vi "Add Monitor Recorders.vi"(6 "Reset":bool, 8 "error in (no error)":errorcluster, 10 "Module type":T1, 11 "Monitor-Pulse in":refnum<class "Application Controller.lvclass">) -> (0 "error out":errorcluster, 2 "Actot names out":string[](array[string]), 3 "Monitor-Pulse out":refnum<class "Application Controller.lvclass">)   [LabVIEW 2018, in "Application Controller.lvclass"]
uses:
  Application Controller.lvclass
  Module Types.ctl
  Instrument Actor/Instrument Actor.lvclass
  C:/github/2018/LabActor/Worker/Worker.lvclass
  Recorders/Micron Optics/Micron Optics Recorder.lvclass
  C:/github/2018/LabActor/Recorders/Spectrometer/Spectrometer.lvclass
  NHMFL_Core/Libraries/Instruments/Micron Optics/Micron Hyperion Driver/Micron Hyperion Driver.lvclass
  C:/github/2018/NHMFL_Core/Libraries/Instruments/Spectrometer Driver/Spectrometer Driver.lvclass
  Spectrum Recorder too/Spectrum Recorder too.lvclass
  C:/github/2018/LabActor/Instrument Actor/Instrument Actor.lvclass
  NHMFL_Core/Libraries/Red Pitaya/RP Core/Red Pitaya Transceiver Driver/Red Pitaya Transceiver Driver.lvclass
  C:/github/2018/NHMFL_Core/Libraries/Instruments/Instrument Driver/Instrument Driver.lvclass
  Instrument Actor/Instrument Actor.lvclass/Instrument Actor.ctl
  Post-Processors/Elastic Moduli/Format Resonances.lvclass
  Application Controller.lvclass/Application Controller.ctl
  Instrument Actor/Write Instrument driver.vi
  Read Monitor ref.vi
  Write Monitor ref.vi
  Worker/Worker.lvclass
  C:/github/2018/LabActor/Template Module/Template Module.lvclass
  Recorders/Spectrometer/Write Spectrometer Driver.lvclass.vi
  NHMFL_Core/Libraries/Queued Listbox/Queued Listbox.xctl
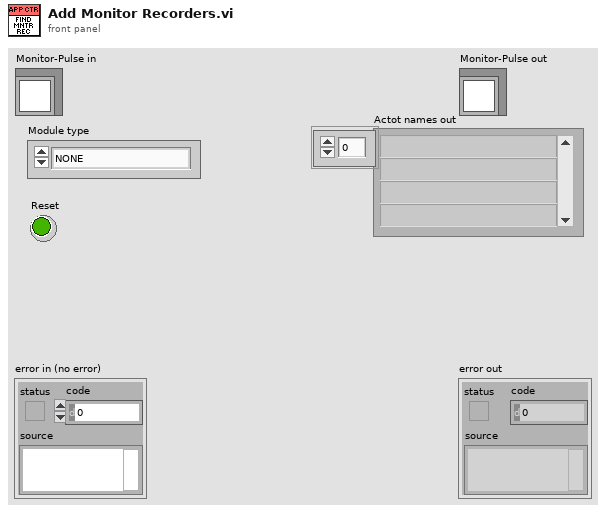
[diagram p1: front panel]
types:
  T1 = typedef "Module Types.ctl" = enum16{"NONE", "NI-DAQmx", "NI-Scope", "Red Pitaya Digitizer", "GaGe", "VISA Device", "Red Pitaya Lockin", "Monitor Controller", "Pulse Controller", "Integrate Pulse", "Lockin Processor", "File converter", "NHMFL Synthesizer", "Micron Hyperion", "Spectrum Recorder", "Resonance Detector", "TCP Communications", "Format Resonances", "Ruby Spectra", "PID Controller"}
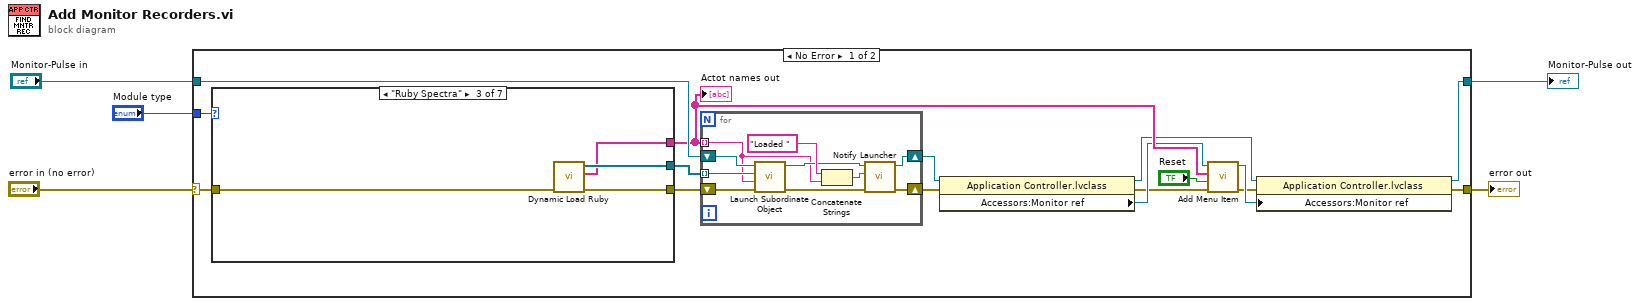
[diagram p0: block diagram]
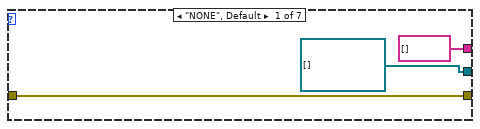
[diagram p2: hidden frame]
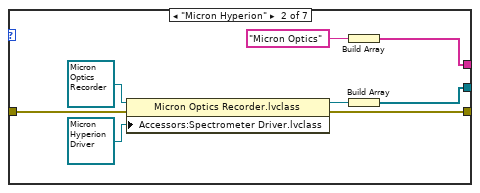
[diagram p3: hidden frame]
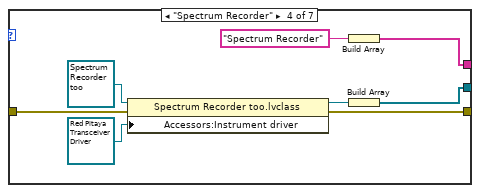
[diagram p4: hidden frame]
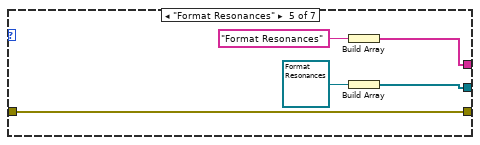
[diagram p5: hidden frame]
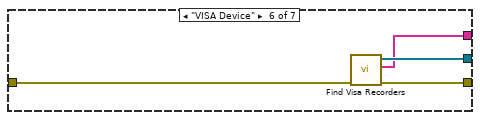
[diagram p6: hidden frame]
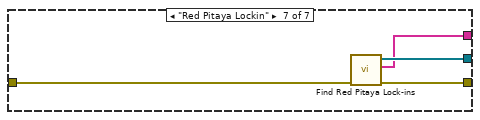
[diagram p7: hidden frame]
diagram:
  n1 = case shown="No Error" "error in (no error)" {
    selector: "error in (no error)" -> [w21 w69]
    tunnel: [w6 w69] -> w4
    tunnel: [w12 w68] -> w2
    tunnel: "Monitor-Pulse in" -> [w20 w68]
    tunnel: "Module type" -> [w17 _]
    frame No Error {
      n2 = case shown="\"Ruby Spectra\"" w17 {
        tunnel: w21 -> [w22 w31 w36 w43 w48 w53 w56]
        tunnel: [refnum<class "Instrument Actor.lvclass">[] [] ("Recorders List") w32 w34 w44 w49 w52 w55] -> w19
        tunnel: [string[] [] ("Names") w25 w33 w37 w45 w51 w54] -> w15
        tunnel: [w22 w30 w35 w42 w48 w50 w57] -> w18
        frame "NONE", Default {
        }
        frame "Micron Hyperion" {
          n3 = property class="Micron Optics Recorder.lvclass"(reference=refnum<class "Micron Optics Recorder.lvclass"> refnum ("Micron Optics Recorder.lvclass"), error in=w31, "Accessors:Spectrometer Driver.lvclass"=refnum<class "Micron Hyperion Driver.lvclass"> refnum ("Micron Hyperion Driver.lvclass")) -> (reference out=w28:refnum<class "Micron Optics Recorder.lvclass">, error out=w30:errorcluster)
          n4 = Build Array("Micron Optics") -> (w25:string[])
          n5 = Build Array(w28) -> (w32:refnum<class "Micron Optics Recorder.lvclass">[])
        }
        frame "Ruby Spectra" {
          n6 = call "Dynamic Load Ruby.vi"("Error In"=w36) -> ("Error Out"=w35:errorcluster, "Device names"=w33:string[], "Digitizers out"=w34:refnum<class "Instrument Actor.lvclass">[])  [unwired: 8 in]
        }
        frame "Spectrum Recorder" {
          n7 = property class="Spectrum Recorder too.lvclass"(reference=refnum<class "Spectrum Recorder too.lvclass"> refnum ("Spectrum Recorder too.lvclass"), error in=w43, "Accessors:Instrument driver"=refnum<class "Red Pitaya Transceiver Driver.lvclass"> refnum ("Red Pitaya Transceiver Driver.lvclass")) -> (reference out=w40:refnum<class "Spectrum Recorder too.lvclass">, error out=w42:errorcluster)
          n8 = Build Array("Spectrum Recorder") -> (w37:string[])
          n9 = Build Array(w40) -> (w44:refnum<class "Spectrum Recorder too.lvclass">[])
        }
        frame "Format Resonances" {
          n10 = Build Array("Format Resonances") -> (w45:string[])
          n11 = Build Array(refnum<class "Format Resonances.lvclass"> refnum ("Elastic Moduli.lvclass")) -> (w49:refnum<class "Format Resonances.lvclass">[])
        }
        frame "VISA Device" {
          n12 = call "Find Visa Recorders.vi"("Error In"=w53) -> ("Error Out"=w50:errorcluster, "Names"=w51:string[], "Recorders List"=w52:refnum<class "Instrument Actor.lvclass">[])  [unwired: 8 in]
        }
        frame "Red Pitaya Lockin" {
          n13 = call "Find Red Pitaya Lock-ins.vi"("Error In"=w56) -> ("Error Out"=w57:errorcluster, "Names"=w54:string[], "Instruments out"=w55:refnum<class "Instrument Actor.lvclass">[])  [unwired: 7 in, 1 out]
        }
      }
      "Actot names out" <- w15
      n14 = for {
        shift-right: [w61] -> w16
        shift-left: w20 -> [w67]
        shift-right: [w59] -> w9
        shift-left: w18 -> [w66]
        tunnel: w19 -> [w65] mode=indexing
        tunnel: w15 -> [w58] mode=indexing
        n15 = call-dynamic "Launch Subordinate Object.vi"("error in (no error)"=w66, "Name"=w58, "Subordinate Object"=w65, "Measure Object in"=w67) -> ("error out"=w60:errorcluster, "Measure Object out"=w62:refnum<class "Application Controller.lvclass">)  [unwired: 5 in, 1 out]
        n16 = Concatenate Strings("Loaded " ("string"), w58) -> (w63:string)
        n17 = call-dynamic "Notify Launcher.vi"("error in (no error)"=w60, "Notification"=w63, "Application Controller in"=w62) -> ("error out"=w59:errorcluster, "Application Controller out"=w61:refnum<class "Application Controller.lvclass">)  [unwired: 7 in]
      }
      n18 = property class="Application Controller.lvclass"(reference=w16, error in=w9) -> (reference out=w13:refnum<class "Application Controller.lvclass">, error out=w8:errorcluster, "Accessors:Monitor ref"=w11:refnum<vi>)
      n19 = call "Add Menu Item.vi"("error in (no error)"=w8, "Reset"="Reset", "Item Names"=w15, "Queed Listbox ref"=w11) -> ("error out"=w7:errorcluster, "Queed Listbox ref out"=w10:refnum<vi>)  [unwired: 5 in, 1 out]
      n20 = property class="Application Controller.lvclass"(reference=w13, error in=w7, "Accessors:Monitor ref"=w10) -> (reference out=w12:refnum<class "Application Controller.lvclass">, error out=w6:errorcluster)
    }
    frame Error {
    }
  }
  "error out" <- w4
  "Monitor-Pulse out" <- w2
